vi "Set Temp of Valve.vi"() -> ()   [LabVIEW 2009]
panel:
  in  "Temp Setting":dbl
  out "Output Value (0)":i32
  out "dup VISA session":refnum<visa-resource-name>
  out "error out":errorcluster
  in  "error in (no error)":errorcluster
  in  "VISA session":refnum<visa-resource-name>
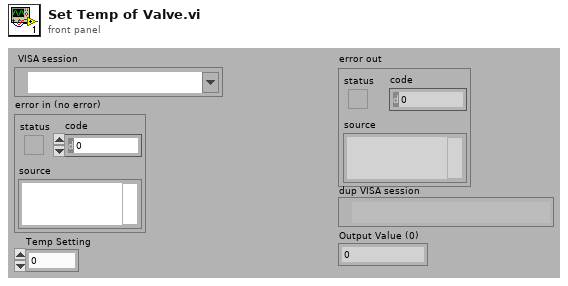
[diagram p1: front panel]
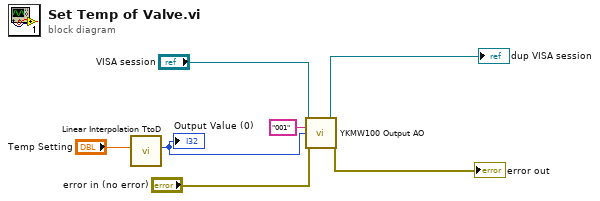
[diagram p0: block diagram]
diagram:
  n1 = call "Linear Interpolation TtoD.vi"("Interp. X"="Temp Setting") -> ("Output Y"=w2:i32)  [unwired: 10 in]
  "Output Value (0)" <- w2
  n2 = call <instrlib>:"YKMW100 Output AO.vi"("VISA session"="VISA session", "Channel String (001)"="001", "Output Value (0)"=w2, "error in (no error)"="error in (no error)") -> ("dup VISA session"=→"dup VISA session":refnum<visa-resource-name>, "error out"=→"error out":errorcluster)  [unwired: 10 in]
